vi "JSON Key to Array Index.vi"(11 "Key":string) -> (1 "Append?":bool, 2 "Is Index?":bool, 3 "Index":i32)   [LabVIEW 2019, in "labview_json.lvlib"]
uses:
  labview_json.lvlib
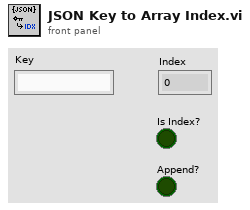
[diagram p1: front panel]
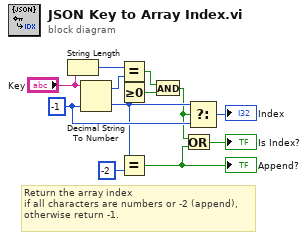
[diagram p0: block diagram]
diagram:
  w8 = -1 ("default (0 I32)")
  # "Return the array index\nif all characters are numbers or -2 (append),\notherwise return -1."
  n1 = String Length(string="Key") -> (length=w11:i32)
  n2 = Decimal String To Number(string="Key", default (0L)=w8) -> (offset past number=w10:i32, number=w5:i32)  [unwired: 1 in]
  n3 = Equal?(x=w11, y=w10) -> (x = y?=w9:bool)
  n4 = Greater Or Equal To 0?(x=w5) -> (x >= 0?=w6:bool)
  n5 = Equal?(x=w5, y=-2) -> (x = y?=w3:bool)
  "Append?" <- w3
  n6 = And(x=w9, y=w6) -> (x .and. y?=w2:bool)
  n7 = Or(x=w2, y=w3) -> (x .or. y?=→"Is Index?":bool)
  n8 = Select(t=w5, s=w2, f=w8) -> (s? t:f=→"Index":i32)
